vi "pco.labview_Live_SoftTrigger_Example.vi"() -> ()   [LabVIEW 2019]
doc: "A short program to demonstrate the fundamentals of control and image acquision with the pco.camera series. The program records a sequence of images, with \"live\" updating, until the \"StopRecording\" button is pressed. Use ctrl-H for more help on the individual controls and indicators.\n\nCopyright 2004, 2010 The Cooke Corporation."
uses:
  pco.sdk/CameraAccess/CameraAccess.lvlib
  pco.sdk/ImageSensor/ImageSensor.lvlib
  pco.sdk/TimingControl/TimingControl.lvlib
  pco.recorder/Recorder.lvlib
  pco.sdk/RecordingControl/RecordingControl.lvlib
  pco.sdk/CameraDescription/CameraDescription.lvlib
  pco.sdk/GeneralCameraControl/GeneralCameraControl.lvlib
panel:
  in  "Trigger":bool
  out "Recorded Images":u32
  in  "Quit":bool
  out "Image":u16[][](graph)
  out "Error":errorcluster {"code" format="%x"}
  in  "Stop Record":bool
  out "Recording On":bool
  in  "roiY1":u16=2 min=2 step=1
  in  "roiX1":u16=2 min=2 step=1
  in  "roiY0":u16=1 min=1 step=1
  in  "roiX0":u16=1 min=1 step=1
  out "Image Height":u16
  out "Image Width":u16
  in  "Image Index":u32 max=9
  in  "dwImgCount":u32=10 caption="Required Number of Images" max=2614
  in  "DelayTimeBase":u16(ring)=2 items=["nanoseconds", "microseconds", "milliseconds"]
  in  "ExposureTimeBase":u16(ring)=2 items=["nanoseconds", "microseconds", "milliseconds"]
  in  "Exposure":u32=10 min=1
  in  "Delay":u32
  in  "Rate":i32(ring) items=["Low", "High"]
  # "This example demonstrates the image acquisition with one camera in ring buffer mode together with a live display of the latest images during record. Here the trigger mode is explicitly set to soft trigger and the Trigger button always forces one image to be acquired\nAfter record is stopped, the images can be addressed by index.\nNote that this example will not be fail save, i.e. doesnt react on errors, just handles them forward to the end\n\nUsage:\nSelect your required image count and the camera setup before you start the program.\nOnce started, the camera will be opened, the recorder will be created, initialized and recording is started.\nBy pressing Trigger a new image is acquired and displayed automatically\nYou can stop the images by pressing stop record.\nAfter stopped, the image at the selected index will be read out\nTo finish the program click on quit application, this will force free and delete of the recorder and a close camera\nYou can change your required ROI after and also during the record."
  # "pco.labview"
  # "Camera Setup"
  # "Recording Control"
  # "Parameters for image readout"
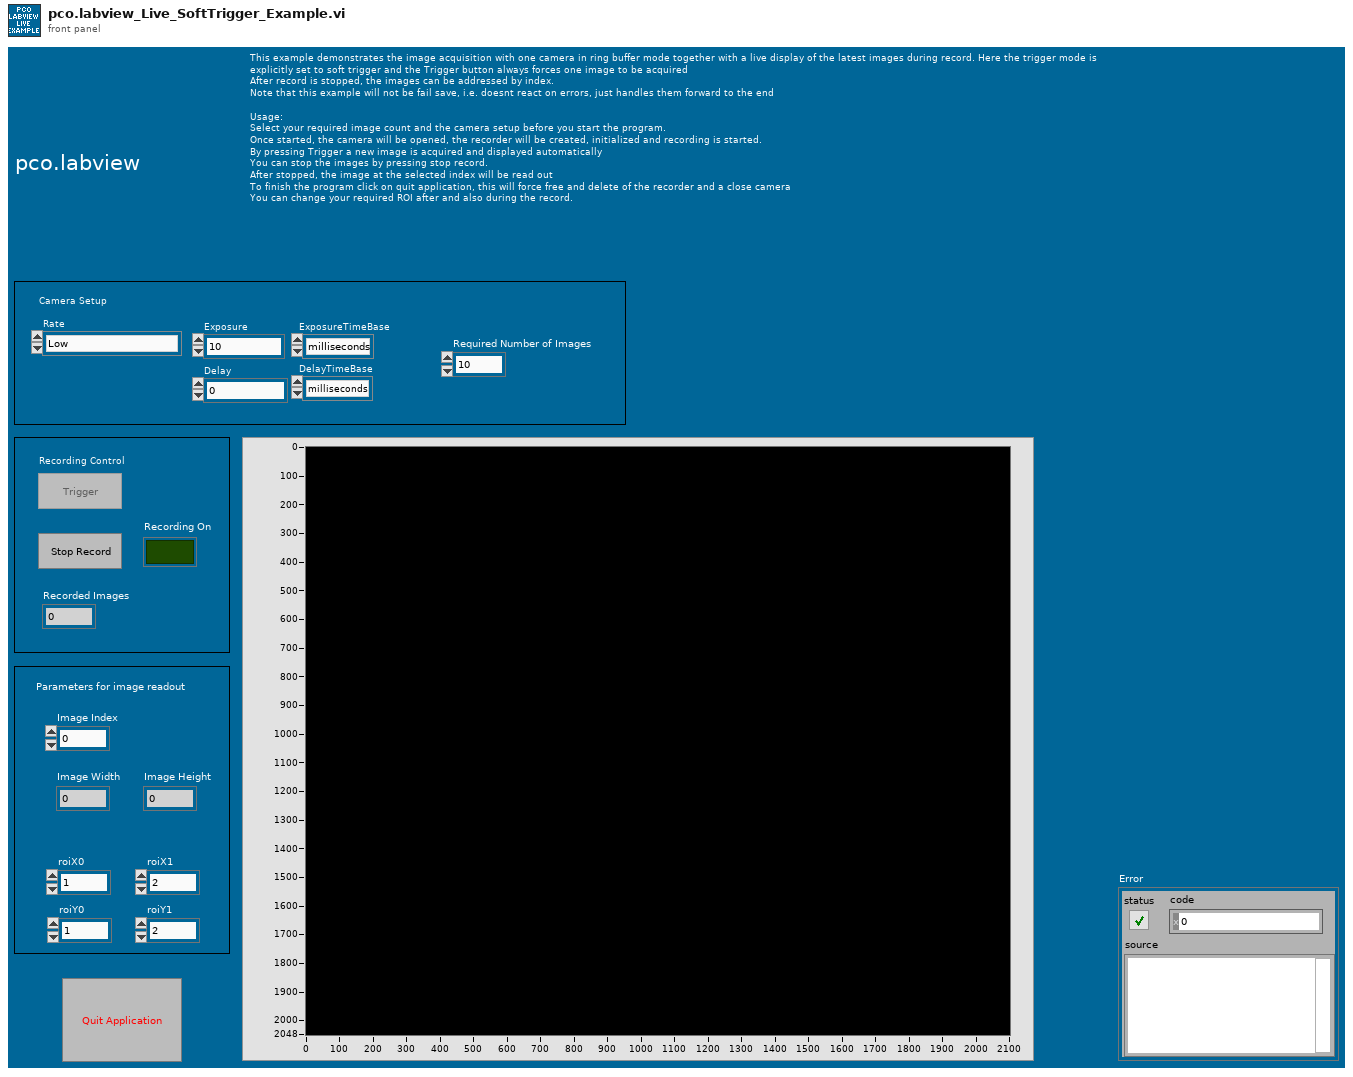
[diagram p1: front panel]
types:
  T1 = enum8{"Enabled", "Disabled", "Disabled and Grayed Out"}
  T2 = cluster{"wSensorTypeDESC":u16, "wSensorSubTypeDESC":u16, "wMaxHorzResStdDESC":u16, "wMaxVertResStdDESC":u16, "wMaxHorzResExtDESC":u16, "wMaxVertResExtDESC":u16, "wDynResDESC":u16, "wMaxBinHorzDESC":u16, "wBinHorzSteppingDESC":u16, "wMaxBinVertDESC":u16, "wBinVertSteppingDESC":u16, "wRoiHorStepsDESC":u16, "wRoiVertStepsDESC":u16, "wNumADCsDESC":u16, "wMinSizeHorzDESC":u16, "dwPixelRateDESC":u32[], "wConvFactDESC":u16[], "sCoolingSetpoints":i16[], "wSoftRoiHorStepsDESC":u16, "wSoftRoiVertStepsDESC":u16, "wIRDESC":u16, "wMinSizeVertDESC":u16, "dwMinDelayDESC":u32, "dwMaxDelayDESC":u32, "dwMinDelayStepDESC":u32, "dwMinExposureDESC":u32, "dwMaxExposureDESC":u32, "dwMinExposureStepDESC":u32, "dwMinDelayIRDESC":u32, "dwMaxDelayIRDESC":u32, "dwMinExposureIRDESC":u32, "dwMaxExposureIRDESC":u32, "wTimeTableDESC":u16, "wDoubleImageDESC":u16, "sMinCoolSetDESC":i16, "sMaxCoolSetDESC":i16, "sDefaultCoolSetDESC":i16, "wPowerDownModeDESC":u16, "wOffsetRegulationDESC":u16, "wColorPatternDESC":u16, "wPatternTypeDESC":u16, "wNumCoolingSetpoints":u16, "dwGeneralCapsDESC1":u32, "dwGeneralCapsDESC2":u32, "dwExtSyncFrequency":u32[], "dwGeneralCapsDESC3":u32, "dwGeneralCapsDESC4":u32}
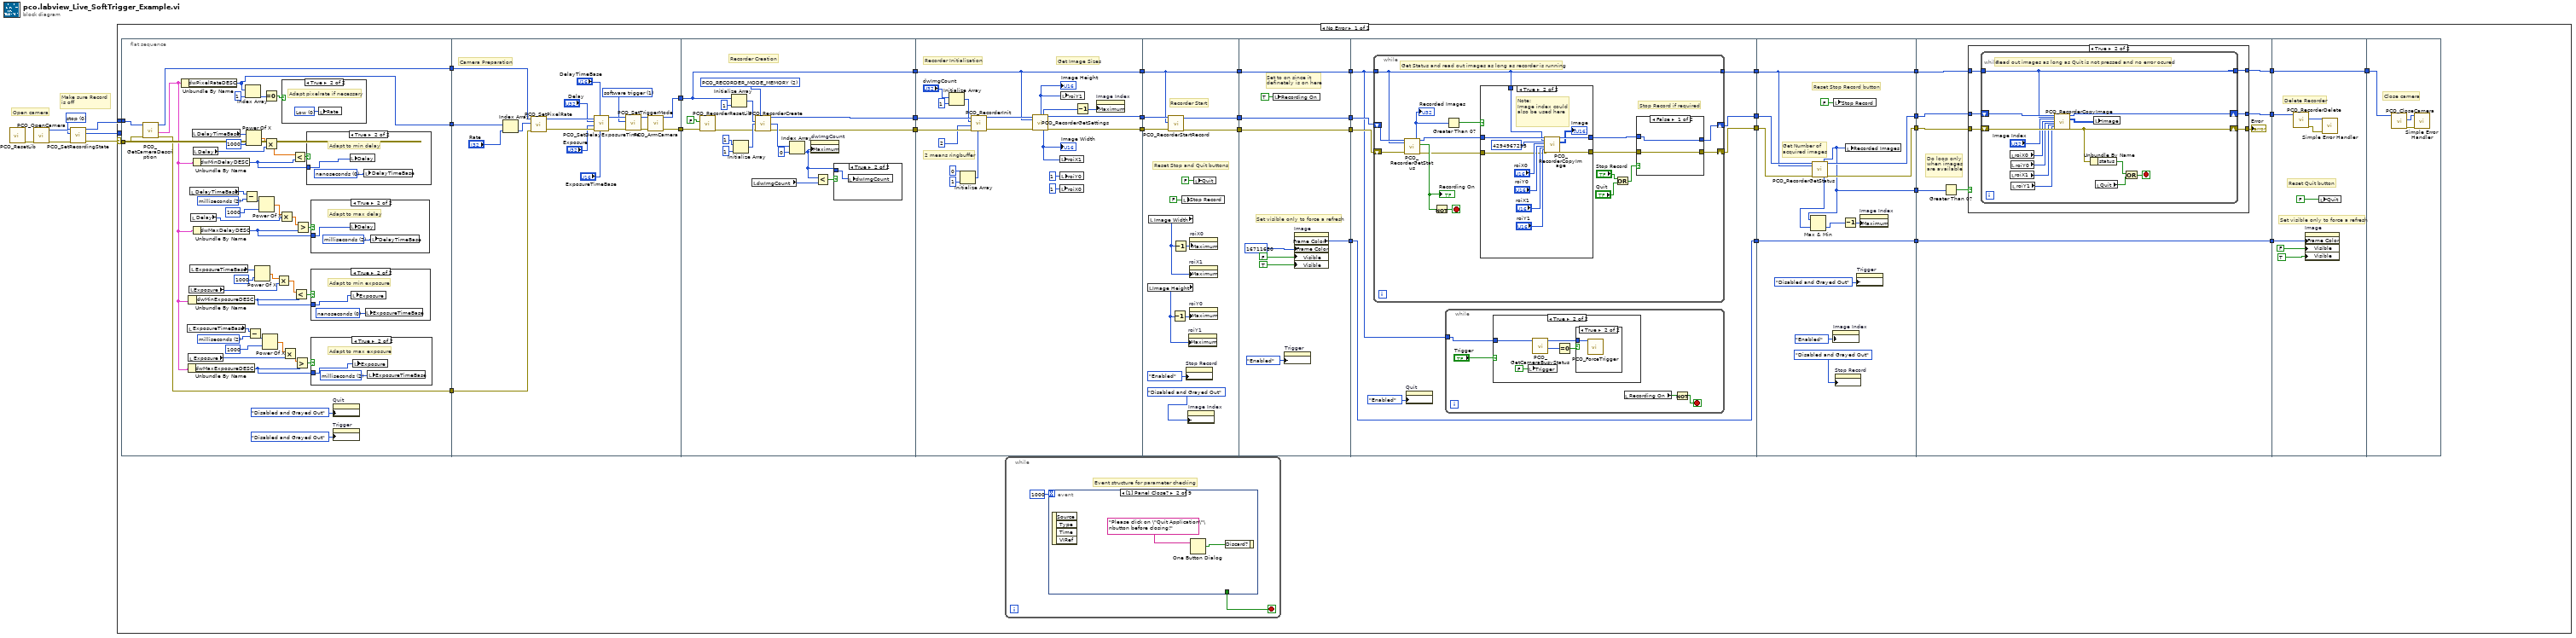
[diagram p0: block diagram]
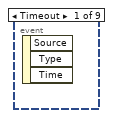
[diagram p2: hidden frame]
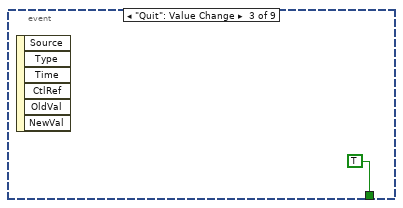
[diagram p3: hidden frame]
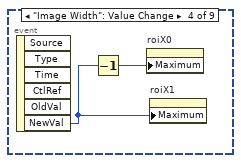
[diagram p4: hidden frame]
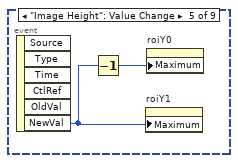
[diagram p5: hidden frame]
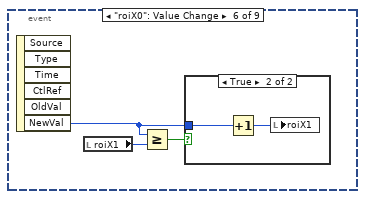
[diagram p6: hidden frame]
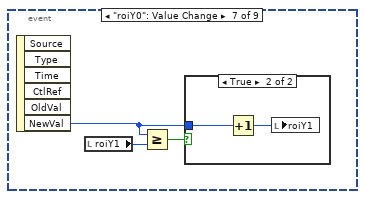
[diagram p8: hidden frame]
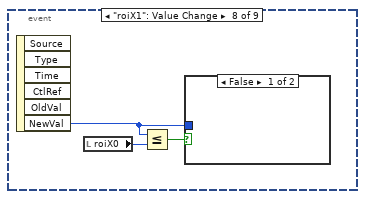
[diagram p10: hidden frame]
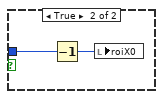
[diagram p11: hidden frame]
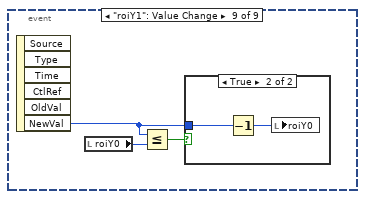
[diagram p12: hidden frame]
diagram:
  w4 = u16 0 items=["stop", "run"] ("wRecState")
  # "Make sure Record \nis off"
  # "Open camera"
  n1 = call "PCO_ResetLib.vi"() -> ("error out"=w7:errorcluster)  [unwired: 10 in, 1 out]
  n2 = call "PCO_OpenCamera.vi"("error in (no error)"=w7) -> ("error out"=w6:errorcluster, "ph out"=w5:u64)  [unwired: 8 in, 1 out]
  n3 = call "PCO_SetRecordingState.vi"("error in (no error)"=w6, "wRecState"=w4, "ph"=w5) -> ("error out"=w2:errorcluster, "ErrorMessage"=w1:i32, "ph out"=w3:u64)  [unwired: 6 in]
  n4 = case shown="No Error" w2 {
    selector: w2 -> [w39 w312]
    tunnel: w3 -> [w40 _]
    tunnel: w1 -> [_ w311]
    frame No Error {
      n5 = flat-sequence {
        tunnel: w39 -> [w109]
        tunnel: w40 -> [w110]
        tunnel: [w104] -> w12
        tunnel: [w112] -> w11
        tunnel: [w111] -> w10
        tunnel: [w122] -> w38
        tunnel: [w123] -> w37
        tunnel: w12 -> [w129]
        tunnel: w11 -> [w128]
        tunnel: w10 -> [w127]
        tunnel: w38 -> [w155]
        tunnel: w37 -> [w144]
        tunnel: [w146] -> w36
        tunnel: [w145] -> w35
        tunnel: [w144] -> w32
        tunnel: w36 -> [w177]
        tunnel: w35 -> [w176]
        tunnel: [w167] -> w34
        tunnel: [w168] -> w33
        tunnel: w32 -> [w166]
        tunnel: [w166] -> w31
        tunnel: w34 -> [w188]
        tunnel: w33 -> [w187]
        tunnel: [w186] -> w22
        tunnel: [w185] -> w20
        tunnel: w31 -> [w184]
        tunnel: [w184] -> w18
        tunnel: w22 -> [w193]
        tunnel: [w193] -> w21
        tunnel: w20 -> [w194]
        tunnel: [w194] -> w19
        tunnel: w18 -> [w195]
        tunnel: [w195] -> w17
        tunnel: [w196] -> w16
        tunnel: w21 -> [w207]
        tunnel: w19 -> [w206]
        tunnel: w17 -> [w200]
        tunnel: [w205] -> w29
        tunnel: [w204] -> w28
        tunnel: [w203] -> w26
        tunnel: w16 -> [w201]
        tunnel: [w201] -> w15
        tunnel: [w260] -> w30
        tunnel: w29 -> [w262]
        tunnel: w28 -> [w263]
        tunnel: [w261] -> w27
        tunnel: w26 -> [w261]
        tunnel: w15 -> [w265]
        tunnel: [w265] -> w13
        tunnel: [w259] -> w9
        tunnel: [w253] -> w8
        tunnel: w30 -> [w275]
        tunnel: w27 -> [w273]
        tunnel: [w271] -> w25
        tunnel: [w270] -> w24
        tunnel: [w269] -> w14
        tunnel: w13 -> [w269]
        tunnel: w9 -> [w274]
        tunnel: w8 -> [w267]
        tunnel: w25 -> [w306]
        tunnel: w24 -> [w303]
        tunnel: [w303] -> w23
        tunnel: w14 -> [w300]
        tunnel: w23 -> [w310]
        frame #0 {
          w71 = u16 2 items=["nanoseconds", "microseconds", "milliseconds"] ("DelayTimeBase")
          w74 = u16 2 items=["nanoseconds", "microseconds", "milliseconds"] ("DelayTimeBase")
          n6 = call "PCO_GetCameraDescription.vi"("error in (no error)"=w109, "ph"=w110) -> ("error out"=w112:errorcluster, "strDescription"=w70:T2, "ph out"=w111:u64)  [unwired: 6 in, 1 out]
          n7 = Unbundle By Name(w70) -> ("dwPixelRateDESC"=w104:u32[])
          n8 = local read "ExposureTimeBase"() -> (w72:u16)
          n9 = Unbundle By Name(w70) -> ("dwMaxExposureDESC"=w101:u32)
          n10 = Unbundle By Name(w70) -> ("dwMinExposureDESC"=w100:u32)
          n11 = local read "Exposure"() -> (w79:u32)
          n12 = local read "Exposure"() -> (w77:u32)
          n13 = local read "DelayTimeBase"() -> (w73:u16)
          n14 = local read "ExposureTimeBase"() -> (w92:u16)
          n15 = local read "Delay"() -> (w84:u32)
          n16 = local read "DelayTimeBase"() -> (w99:u16)
          n17 = local read "Delay"() -> (w95:u32)
          n18 = Unbundle By Name(w70) -> ("dwMinDelayDESC"=w97:u32)
          n19 = Unbundle By Name(w70) -> ("dwMaxDelayDESC"=w102:u32)
          n20 = Subtract(x=w73, y=w74) -> (x-y=w88:i32)
          n21 = Index Array(array=w104, index=1) -> (element=w106:u32)
          n22 = Power Of X(1:u32 1000 ("Delay"), 2:w99) -> (0:w96:dbl)
          n23 = Subtract(x=w72, y=w71) -> (x-y=w80:i32)
          n24 = Power Of X(1:u32 1000 ("Delay"), 2:w92) -> (0:w91:dbl)
          n25 = Power Of X(1:u32 1000 ("Delay"), 2:w88) -> (0:w85:dbl)
          n26 = Power Of X(1:u32 1000 ("Delay"), 2:w80) -> (0:w82:dbl)
          n27 = Equal To 0?(x=w106) -> (x = 0?=w105:bool)
          n28 = Multiply(x=w96, y=w95) -> (x*y=w94:dbl)
          n29 = Multiply(x=w91, y=w77) -> (x*y=w76:dbl)
          n30 = Multiply(x=w85, y=w84) -> (x*y=w86:dbl)
          n31 = case shown="True" w105 {
            frame False {
            }
            frame True {
              w121 = 0 items=["Low", "High"] ("Rate")
              # "Adapt pixelrate if necessary"
              n32 = local write "Rate"(w121) -> ()
            }
          }
          n33 = Multiply(x=w82, y=w79) -> (x*y=w78:dbl)
          n34 = Less?(x=w94, y=w97) -> (x < y?=w93:bool)
          n35 = Less?(x=w76, y=w100) -> (x < y?=w75:bool)
          n36 = Greater?(x=w78, y=w101) -> (0:w83:bool)
          n37 = Greater?(x=w86, y=w102) -> (0:w89:bool)
          n38 = case shown="True" w93 {
            tunnel: w97 -> [_ w120]
            frame False {
            }
            frame True {
              w119 = u16 0 items=["nanoseconds", "microseconds", "milliseconds"] ("DelayTimeBase")
              # "Adapt to min delay"
              n39 = local write "Delay"(w120) -> ()
              n40 = local write "DelayTimeBase"(w119) -> ()
            }
          }
          n41 = case shown="True" w89 {
            tunnel: w102 -> [_ w118]
            frame False {
            }
            frame True {
              w117 = u16 2 items=["nanoseconds", "microseconds", "milliseconds"] ("DelayTimeBase")
              # "Adapt to max delay"
              n42 = local write "Delay"(w118) -> ()
              n43 = local write "DelayTimeBase"(w117) -> ()
            }
          }
          n44 = case shown="True" w75 {
            tunnel: w100 -> [_ w116]
            frame False {
            }
            frame True {
              w115 = u16 0 items=["nanoseconds", "microseconds", "milliseconds"] ("DelayTimeBase")
              # "Adapt to min exposure"
              n45 = local write "Exposure"(w116) -> ()
              n46 = local write "ExposureTimeBase"(w115) -> ()
            }
          }
          n47 = case shown="True" w83 {
            tunnel: w101 -> [_ w114]
            frame False {
            }
            frame True {
              w113 = u16 2 items=["nanoseconds", "microseconds", "milliseconds"] ("DelayTimeBase")
              # "Adapt to max exposure"
              n48 = local write "Exposure"(w114) -> ()
              n49 = local write "ExposureTimeBase"(w113) -> ()
            }
          }
          n50 = property on="Quit" class="Bool (strict)"("DisabledEnum"=T1."Disabled and Grayed Out" ("Disabled")) -> ()  [unwired: 2 in, 2 out]
          n51 = property on="Trigger" class="Bool (strict)"("DisabledEnum"=T1."Disabled and Grayed Out" ("Disabled")) -> ()  [unwired: 2 in, 2 out]
        }
        frame #1 {
          w126 = u16 1 items=["auto sequence"=0, "software trigger"=1, "external exposure start & software trigger"=2, "external exposure control"=3, "external synchronized"=4, "fast external exposure control"=5, "external CDS control"=6, "slow external exposure control"=7, "external synchronized HDSDI"=258] ("wTriggerMode")
          # "Camera Preparation"
          n52 = Index Array(array=w129, index="Rate") -> (element=w138:u32)
          n53 = call "PCO_SetPixelRate.vi"("error in (no error)"=w128, "dwPixelRate"=w138, "ph"=w127) -> ("error out"=w136:errorcluster, "ph out"=w137:u64)  [unwired: 6 in, 1 out]
          n54 = call "PCO_SetDelayExposureTime.vi"("wTimeBaseExposure"="ExposureTimeBase", "wTimeBaseDelay"="DelayTimeBase", "error in (no error)"=w136, "dwExposure"="Exposure", "dwDelay"="Delay", "ph"=w137) -> ("error out"=w130:errorcluster, "ph out"=w131:u64)  [unwired: 3 in, 1 out]
          n55 = call "PCO_SetTriggerMode.vi"("error in (no error)"=w130, "wTriggerMode"=w126, "ph"=w131) -> ("error out"=w124:errorcluster, "ph out"=w125:u64)  [unwired: 6 in, 1 out]
          n56 = call "PCO_ArmCamera.vi"("error in (no error)"=w124, "ph"=w125) -> ("error out"=w122:errorcluster, "ph out"=w123:u64)  [unwired: 7 in, 1 out]
        }
        frame #2 {
          w140 = u16 2 items=["PCO_RECORDER_MODE_FILE"=1, "PCO_RECORDER_MODE_MEMORY"=2, "PCO_RECORDER_MODE_CAMRAM"=3] ("dwRecMode")
          # "Recorder Creation"
          n57 = call "PCO_RecorderResetLib.vi"("error in (no error)"=w155, "bSilent"=FALSE) -> ("error out"=w147:errorcluster)  [unwired: 8 in, 1 out]
          n58 = Initialize Array(w144, 1 ("dimension size")) -> (w153:u64[])
          n59 = Initialize Array(u32 1 ("dimension size"), 1 ("dimension size")) -> (w150:u32[])
          n60 = local read "dwImgCount"() -> (w141:u32)
          n61 = call "PCO_RecorderCreate.vi"("wRecMode"=w140, "phCamArr"=w153, "dwImgDistributionArr"=w150, "error in (no error)"=w147) -> ("phRec out"=w145:u64, "dwMaxImgCountArr"=w149:u32[], "error out"=w146:errorcluster)  [unwired: 8 in, 1 out]
          n62 = Index Array(array=w149, index=0) -> (element=w142:u32)
          n63 = property on="dwImgCount" class="DigNum (strict)"("Maximum"=w142) -> ()  [unwired: 2 in, 2 out]
          n64 = Less?(x=w142, y=w141) -> (x < y?=w143:bool)
          n65 = case shown="True" w143 {
            tunnel: w142 -> [_ w157]
            frame False {
            }
            frame True {
              n66 = local write "dwImgCount"(w157) -> ()
            }
          }
        }
        frame #3 {
          # "2 means ringbuffer"
          # "Get Image Sizes"
          # "Recorder Initialization"
          n67 = Initialize Array("dwImgCount", 1 ("dimension size")) -> (w173:u32[])
          n68 = Initialize Array(u16 0 ("element"), 1 ("dimension size")) -> (w158:u16[])
          n69 = call "PCO_RecorderInit.vi"("wRamSegmentArr"=w158, "error in (no error)"=w177, "wType"=u16 2, "dwImgCountArr"=w173, "phRec"=w176) -> ("error out"=w172:errorcluster, "phRec out"=w171:u64)  [unwired: 4 in, 1 out]
          n70 = call "PCO_RecorderGetSettings.vi"("phRec"=w171, "phCam"=w166, "error in (no error)"=w172) -> ("wHeight"=w165:u16, "dwReqImgCount"=w162:u32, "phRec out"=w167:u64, "wWidth"=w164:u16, "error out"=w168:errorcluster)  [unwired: 4 in, 4 out]
          "Image Height" <- w165
          "Image Width" <- w164
          n71 = local write "roiX1"(w164) -> ()
          n72 = local write "roiX0"(u16 1 ("roiY0")) -> ()
          n73 = local write "roiY0"(u16 1 ("roiY0")) -> ()
          n74 = local write "roiY1"(w165) -> ()
          n75 = Decrement(x=w162) -> (x-1=w163:u32)
          n76 = property on="Image Index" class="DigNum (strict)"("Maximum"=w163) -> ()  [unwired: 2 in, 2 out]
        }
        frame #4 {
          # "Reset Stop and Quit buttons"
          # "Recorder Start"
          n77 = local read "Image Height"() -> (w181:u16)
          n78 = local read "Image Width"() -> (w180:u16)
          n79 = call "PCO_RecorderStartRecord.vi"("error in (no error)"=w187, "phCam"=w184, "phRec"=w188) -> ("error out"=w186:errorcluster, "phRec out"=w185:u64)  [unwired: 6 in, 1 out]
          n80 = Decrement(x=w181) -> (x-1=w182:u16)
          n81 = Decrement(x=w180) -> (x-1=w183:u16)
          n82 = local write "Stop Record"(FALSE ("Stop Record")) -> ()
          n83 = property on="Stop Record" class="Bool (strict)"("DisabledEnum"=T1."Enabled" ("Disabled")) -> ()  [unwired: 2 in, 2 out]
          n84 = property on="Image Index" class="DigNum (strict)"("DisabledEnum"=T1."Disabled and Grayed Out" ("Disabled")) -> ()  [unwired: 2 in, 2 out]
          n85 = property on="roiY1" class="DigNum (strict)"("Maximum"=w181) -> ()  [unwired: 2 in, 2 out]
          n86 = property on="roiX1" class="DigNum (strict)"("Maximum"=w180) -> ()  [unwired: 2 in, 2 out]
          n87 = property on="roiY0" class="DigNum (strict)"("Maximum"=w182) -> ()  [unwired: 2 in, 2 out]
          n88 = property on="roiX0" class="DigNum (strict)"("Maximum"=w183) -> ()  [unwired: 2 in, 2 out]
          n89 = local write "Quit"(FALSE ("Stop")) -> ()
        }
        frame #5 {
          # "Set to on since it \ndefinetely is on here"
          # "Set visible only to force a refresh"
          n90 = local write "Recording On"(TRUE ("Recording On")) -> ()
          n91 = property on="Trigger" class="Bool (strict)"("DisabledEnum"=T1."Enabled" ("Disabled")) -> ()  [unwired: 2 in, 2 out]
          n92 = property on="Image" class="IntGraph (strict)"("Frame Color"=u32 16711680, "Visible"=FALSE, "Visible"=TRUE) -> ("Frame Color"=w196:u32)  [unwired: 2 in, 2 out]
        }
        frame #6 {
          n93 = while {
            tunnel: w200 -> [w212]
            shift-right: [w213] -> w204
            shift-left: w207 -> [w223]
            shift-right: [w214] -> w205
            shift-left: w206 -> [w219]
            tunnel: [w212] -> w203
            stop <- w218 stop-if-true
            # "Stop Record if required"
            # "Get Status and read out images as long as recorder is running"
            n94 = call "PCO_RecorderGetStatus.vi"("phRec"=w219, "phCam"=w212, "error in (no error)"=w223) -> ("dwProcImgCount"=w209:u32, "phRec out"=w221:u64, "bIsRunning"=w222:bool, "error out"=w220:errorcluster)  [unwired: 5 in, 8 out]
            "Recording On" <- w222
            "Recorded Images" <- w209
            n95 = Not(x=w222) -> (.not. x?=w218:bool)
            n96 = Greater Than 0?(x=w209) -> (x > 0?=w208:bool)
            n97 = case shown="True" w208 {
              tunnel: w221 -> [w225 w236]
              tunnel: w220 -> [w224 w230]
              tunnel: [w225 w229] -> w217
              tunnel: [w224 w228] -> w216
              tunnel: w212 -> [_ w226]
              frame False {
              }
              frame True {
                # "Note: \nImage index could \nalso be used here"
                n98 = call "PCO_RecorderCopyImage.vi"("phRec"=w236, "phCam"=w226, "dwImgIdx"=u32 4294967295, "wRoiX0"="roiX0", "wRoiY0"="roiY0", "wRoiX1"="roiX1", "wRoiY1"="roiY1", "error in (no error)"=w230) -> ("phRec out"=w229:u64, "wImgBuf"=→"Image":u16[][], "error out"=w228:errorcluster)  [unwired: 13 in, 4 out]
              }
            }
            n99 = Or(x="Stop Record", y="Quit") -> (x .or. y?=w215:bool)
            n100 = case shown="False" w215 {
              tunnel: w217 -> [w238 w242]
              tunnel: w216 -> [w237 w241]
              tunnel: [w238 w239] -> w214
              tunnel: [w237 w240] -> w213
              frame False {
              }
              frame True {
                n101 = call "PCO_RecorderStopRecord.vi"("error in (no error)"=w241, "phRec"=w242) -> ("error out"=w240:errorcluster, "phRec out"=w239:u64)  [unwired: 7 in, 1 out]
              }
            }
          }
          n102 = property on="Quit" class="Bool (strict)"("DisabledEnum"=T1."Enabled" ("Disabled")) -> ()  [unwired: 2 in, 2 out]
          n103 = while {
            tunnel: w200 -> [w244]
            stop <- w246 stop-if-true
            n104 = case shown="True" "Trigger" {
              tunnel: w244 -> [_ w248]
              frame False {
              }
              frame True {
                n105 = local write "Trigger"(FALSE ("Trigger")) -> ()
                n106 = call "PCO_GetCameraBusyStatus.vi"("ph"=w248) -> ("wCameraBusyState"=w251:u16, "ph out"=w249:u64)  [unwired: 7 in, 2 out]
                n107 = Equal To 0?(x=w251) -> (x = 0?=w250:bool)
                n108 = case shown="True" w250 {
                  tunnel: w249 -> [_ w252]
                  frame False {
                  }
                  frame True {
                    n109 = call "PCO_ForceTrigger.vi"("ph"=w252) -> ()  [unwired: 7 in, 4 out]
                  }
                }
              }
            }
            n110 = local read "Recording On"() -> (w245:bool)
            n111 = Not(x=w245) -> (.not. x?=w246:bool)
          }
        }
        frame #7 {
          # "Get Number of \nacquired images"
          # "Reset Stop Record button"
          n112 = call "PCO_RecorderGetStatus.vi"("phRec"=w262, "phCam"=w261, "error in (no error)"=w263) -> ("dwProcImgCount"=w253:u32, "dwReqImgCount"=w256:u32, "phRec out"=w260:u64, "error out"=w259:errorcluster)  [unwired: 5 in, 8 out]
          n113 = Max & Min(x=w253, y=w256) -> (min(x,y)=w257:u32)  [unwired: 1 out]
          n114 = property on="Image Index" class="DigNum (strict)"("DisabledEnum"=T1."Enabled" ("Disabled")) -> ()  [unwired: 2 in, 2 out]
          n115 = local write "Stop Record"(FALSE ("Stop Record")) -> ()
          n116 = property on="Stop Record" class="Bool (strict)"("DisabledEnum"=T1."Disabled and Grayed Out" ("Disabled")) -> ()  [unwired: 2 in, 2 out]
          n117 = Decrement(x=w257) -> (x-1=w258:u32)
          n118 = local write "Recorded Images"(w253) -> ()
          n119 = property on="Trigger" class="Bool (strict)"("DisabledEnum"=T1."Disabled and Grayed Out" ("Disabled")) -> ()  [unwired: 2 in, 2 out]
          n120 = property on="Image Index" class="DigNum (strict)"("Maximum"=w258) -> ()  [unwired: 2 in, 2 out]
        }
        frame #8 {
          # "Do loop only\nwhen images\nare available"
          n121 = Greater Than 0?(x=w267) -> (x > 0?=w268:bool)
          n122 = case shown="True" w268 {
            tunnel: w275 -> [w278 w285]
            tunnel: w274 -> [w277 w284]
            tunnel: w273 -> [w279 w283]
            tunnel: [w277 w282] -> w272
            tunnel: [w278 w281] -> w271
            tunnel: [w279 w280] -> w270
            frame False {
              n123 = One Button Dialog(message="No Images have been acquired") -> ()  [unwired: 1 in, 1 out]
            }
            frame True {
              n124 = while {
                shift-right: [w287] -> w282
                shift-left: w284 -> [w296]
                shift-right: [w288] -> w281
                shift-left: w285 -> [w295]
                tunnel: w283 -> [w286]
                tunnel: [w286] -> w280
                stop <- w297 stop-if-true
                # "Read out images as long as Quit is not pressed and no error ocured"
                n125 = local read "roiX0"() -> (w293:u16)
                n126 = local read "roiX1"() -> (w291:u16)
                n127 = local read "roiY0"() -> (w292:u16)
                n128 = local read "roiY1"() -> (w290:u16)
                n129 = call "PCO_RecorderCopyImage.vi"("phRec"=w295, "phCam"=w286, "dwImgIdx"="Image Index", "wRoiX0"=w293, "wRoiY0"=w292, "wRoiX1"=w291, "wRoiY1"=w290, "error in (no error)"=w296) -> ("phRec out"=w288:u64, "wImgBuf"=w289:u16[][], "error out"=w287:errorcluster)  [unwired: 13 in, 4 out]
                n130 = Unbundle By Name(w287) -> ("status"=w299:bool)
                n131 = local write "Image"(w289) -> ()
                n132 = local read "Quit"() -> (w298:bool)
                n133 = Or(x=w299, y=w298) -> (x .or. y?=w297:bool)
              }
            }
          }
          "Error" <- w272
        }
        frame #9 {
          # "Set visible only to force a refresh"
          # "Delete Recorder"
          # "Reset Quit button"
          n134 = call "PCO_RecorderDelete.vi"("phRec"=w306) -> ("error out"=w304:errorcluster, "ErrorMessage"=w305:i32)  [unwired: 9 in]
          n135 = property on="Image" class="IntGraph (strict)"("Frame Color"=w300, "Visible"=FALSE, "Visible"=TRUE) -> ()  [unwired: 2 in, 2 out]
          n136 = local write "Quit"(FALSE ("Stop Record")) -> ()
          n137 = call <vilib>:"Simple Error Handler.vi"("error code (no error:0)"=w305, "error in (no error)"=w304) -> ()  [unwired: 3 in, 5 out]
        }
        frame #10 {
          # "Close camera"
          n138 = call "PCO_CloseCamera.vi"("ph"=w310) -> ("error out"=w308:errorcluster, "ErrorMessage"=w309:i32)  [unwired: 9 in]
          n139 = call <vilib>:"Simple Error Handler.vi"("error code (no error:0)"=w309, "error in (no error)"=w308) -> ()  [unwired: 3 in, 5 out]
        }
      }
      n140 = while {
        stop <- w41 stop-if-true
        # "Event structure for parameter checking"
        n141 = event shown="[1] Panel Close?" {
          selector: _ -> [_ _ _ _ _ _ _ _ _]
          dyn-events: _ -> [_ _ _ _ _ _ _ _ _]
          timeout: 1000 -> [_ _ _ _ _ _ _ _ _]
          tunnel: [_ _ TRUE _ _ _ _ _ _] -> w41
          event Timeout {
            n142 = event-data() -> ()  [unwired: 1 in, 3 out]
          }
          event Panel Close? {
            n143 = event-data() -> ()  [unwired: 1 in, 4 out]
            n144 = One Button Dialog(message="Please click on \"Quit Application\"\nbutton before closing!") -> (true=w43:bool)  [unwired: 1 in]
            n145 = event-data("Discard?"=w43) -> ()  [unwired: 1 in, 1 out]
          }
          event "Quit": Value Change {
            n146 = event-data() -> ()  [unwired: 1 in, 6 out]
          }
          event "Image Width": Value Change {
            n147 = event-data() -> ("NewVal"=w46:u16)  [unwired: 1 in, 5 out]
            n148 = Decrement(x=w46) -> (x-1=w47:u16)
            n149 = property on="roiX0" class="DigNum (strict)"("Maximum"=w47) -> ()  [unwired: 2 in, 2 out]
            n150 = property on="roiX1" class="DigNum (strict)"("Maximum"=w46) -> ()  [unwired: 2 in, 2 out]
          }
          event "Image Height": Value Change {
            n151 = event-data() -> ("NewVal"=w48:u16)  [unwired: 1 in, 5 out]
            n152 = Decrement(x=w48) -> (x-1=w49:u16)
            n153 = property on="roiY1" class="DigNum (strict)"("Maximum"=w48) -> ()  [unwired: 2 in, 2 out]
            n154 = property on="roiY0" class="DigNum (strict)"("Maximum"=w49) -> ()  [unwired: 2 in, 2 out]
          }
          event "roiX0": Value Change {
            n155 = event-data() -> ("NewVal"=w50:u16)  [unwired: 1 in, 5 out]
            n156 = local read "roiX1"() -> (w52:u16)
            n157 = Greater Or Equal?(x=w50, y=w52) -> (x >= y?=w51:bool)
            n158 = case shown="True" w51 {
              tunnel: w50 -> [_ w54]
              frame False {
              }
              frame True {
                n159 = Increment(x=w54) -> (x+1=w53:u16)
                n160 = local write "roiX1"(w53) -> ()
              }
            }
          }
          event "roiY0": Value Change {
            n161 = event-data() -> ("NewVal"=w55:u16)  [unwired: 1 in, 5 out]
            n162 = local read "roiY1"() -> (w57:u16)
            n163 = Greater Or Equal?(x=w55, y=w57) -> (x >= y?=w56:bool)
            n164 = case shown="True" w56 {
              tunnel: w55 -> [_ w59]
              frame False {
              }
              frame True {
                n165 = Increment(x=w59) -> (x+1=w58:u16)
                n166 = local write "roiY1"(w58) -> ()
              }
            }
          }
          event "roiX1": Value Change {
            n167 = event-data() -> ("NewVal"=w60:u16)  [unwired: 1 in, 5 out]
            n168 = local read "roiX0"() -> (w62:u16)
            n169 = Less Or Equal?(x=w60, y=w62) -> (x <= y?=w61:bool)
            n170 = case shown="False" w61 {
              tunnel: w60 -> [_ w64]
              frame False {
              }
              frame True {
                n171 = Decrement(x=w64) -> (x-1=w63:u16)
                n172 = local write "roiX0"(w63) -> ()
              }
            }
          }
          event "roiY1": Value Change {
            n173 = event-data() -> ("NewVal"=w65:u16)  [unwired: 1 in, 5 out]
            n174 = local read "roiY0"() -> (w67:u16)
            n175 = Less Or Equal?(x=w65, y=w67) -> (x <= y?=w66:bool)
            n176 = case shown="True" w66 {
              tunnel: w65 -> [_ w69]
              frame False {
              }
              frame True {
                n177 = Decrement(x=w69) -> (x-1=w68:u16)
                n178 = local write "roiY0"(w68) -> ()
              }
            }
          }
        }
      }
    }
    frame Error {
      n179 = call <vilib>:"Simple Error Handler.vi"("error code (no error:0)"=w311, "error in (no error)"=w312) -> ()  [unwired: 3 in, 5 out]
    }
  }
